vi "open standards data 2.vi"(11 "file path":path) -> (0 "canceled":bool, 1 "standard cluster":T1={"Description"="", "Setup"={"integration time"=0.5, "rinse time"=10.0, "sample time"=10.0, "sample type"=0}, "Concentrations"=[], "Absorbance"=[], "Analyst"="", "Concentration units"="", "Good"=[]} {"Absorbance" format="%.2e"; "Concentrations" format="%.3e"; "Setup"."sample type" items=["Sample Cuvet", "Sipper Cell", "No Dialog"]; "Setup"."sample time" min=0.0 max=100.0 step=1.0 format="%.1f"; "Setup"."rinse time" min=0.0 max=100.0 step=1.0 format="%.1f"; "Setup"."integration time" format="%.1f"}, 3 "new file path":path)   [LabVIEW 2015]
uses:
  standard cluster.ctl
  settings.ctl
  file/file action.ctl
panel:
  out "error out":errorcluster
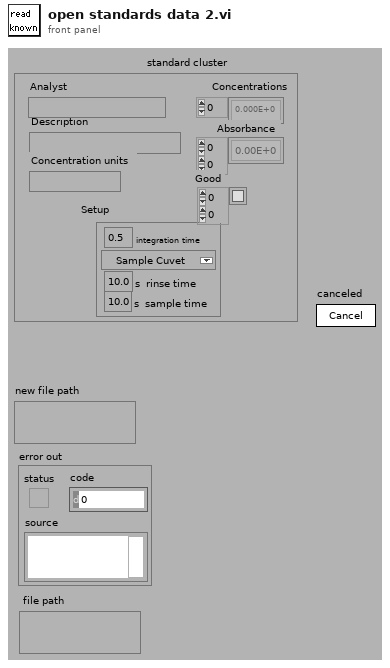
[diagram p1: front panel]
types:
  T1 = typedef "standard cluster.ctl" = cluster{"Description":string, "Setup":T2, "Concentrations":dbl[], "Absorbance":dbl[][], "Analyst":string, "Concentration units":string, "Good":bool[][]}
  T2 = typedef "settings.ctl" = cluster{"integration time":sgl, "rinse time":dbl[unit], "sample time":dbl[unit], "sample type":u16}
  T3 = typedef "file action.ctl" = enum16{"Save", "Open"}
  T4 = enum16{"open", "open or create", "create or replace", "create", "open (read only)"}
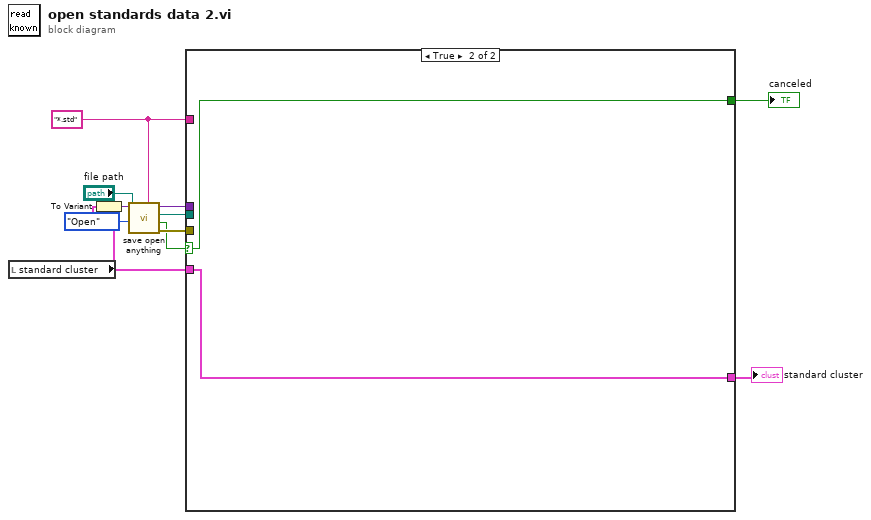
[diagram p0: block diagram]
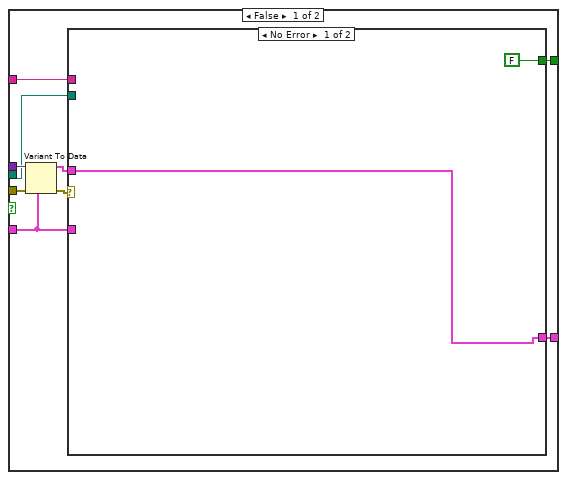
[diagram p2: hidden frame]
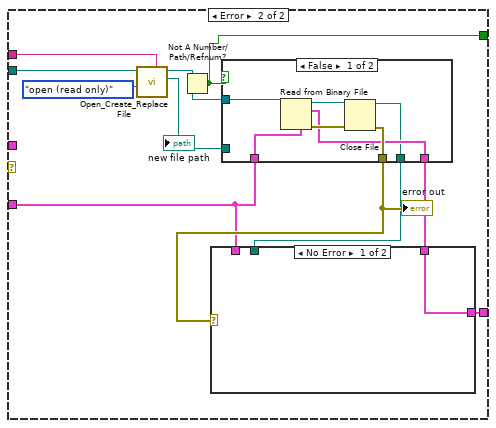
[diagram p3: hidden frame]
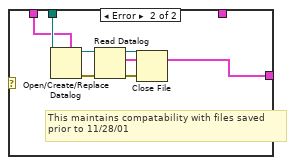
[diagram p4: hidden frame]
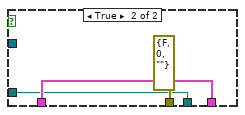
[diagram p5: hidden frame]
diagram:
  w4 = "*.std" ("pattern")
  n1 = local read "standard cluster"() -> (w6:T1)
  n2 = To Variant(anything=w6) -> (Variant=w10:variant)
  n3 = call "save open anything.vi"("Variant"=w10, "file path"="file path", "Action"=file_action."Open", "pattern"=w4) -> ("Variant out"=w8:variant, "new file path"=w5:path, "canceled"=w2:bool, "error out"=w7:errorcluster)  [unwired: 3 in]
  n4 = case shown="True" w2 {
    selector: w2 -> [_ w52]
    tunnel: [w20 w53] -> w11
    tunnel: w8 -> [w19 _]
    tunnel: w7 -> [w18 _]
    tunnel: w6 -> [w17 w53]
    tunnel: w5 -> [w14 _]
    tunnel: w4 -> [w13 _]
    tunnel: [w12 w52] -> w1
    frame False {
      n5 = Variant To Data(error in=w18, type=w17, Variant=w19) -> (data=w15:T1, error out=w16:errorcluster)
      n6 = case shown="No Error" w16 {
        tunnel: [w22 w30] -> w20
        tunnel: w13 -> [_ w26]
        tunnel: w17 -> [_ w25]
        tunnel: w15 -> [w22 _]
        tunnel: w14 -> [_ w24]
        tunnel: [FALSE w23] -> w12
        frame No Error {
        }
        frame Error {
          n7 = call <vilib>:"Open_Create_Replace File.vi"("pattern"=w26, "function (open:0)"=T4."open (read only)", "file path"=w24) -> ("new file path"=w27:path, "refnum"=w32:refnum<file>)  [unwired: 5 in, 2 out]
          "new file path" <- w27
          n8 = Not A Number/Path/Refnum?(number/path/refnum=w32) -> (NaN/Path/Refnum?=w23:bool)
          n9 = case shown="False" w23 {
            tunnel: w32 -> [w46 _]
            tunnel: w25 -> [w45 w50]
            tunnel: [w44 errorcluster {"status"=FALSE, "code"=0, "source"=""} ("error out")] -> w31
            tunnel: [w43 w50] -> w29
            tunnel: [w42 w49] -> w28
            tunnel: w27 -> [_ w49]
            frame False {
              n10 = Read from Binary File(5:w45, 11:w46) -> (0:w47:errorcluster, 2:w43:T1, 3:w48:refnum<file>)  [unwired: 4 in, 1 out]
              n11 = Close File(refnum=w48, error in=w47) -> (path=w42:path, error out=w44:errorcluster)
            }
            frame True {
            }
          }
          "error out" <- w31
          n12 = case shown="No Error" w31 {
            tunnel: [w34 w41] -> w30
            tunnel: w29 -> [w34 _]
            tunnel: w28 -> [_ w36]
            tunnel: w25 -> [_ w35]
            frame No Error {
            }
            frame Error {
              # "This maintains compatability with files saved \nprior to 11/28/01"
              n13 = Open/Create/Replace Datalog(5:w35, 11:w36) -> (0:w38:errorcluster, 3:w39:refnum<k1>)  [unwired: 4 in, 1 out]
              n14 = Read Datalog(4:w38, 7:w39) -> (0:w37:errorcluster, 2:w41:T1, 3:w40:refnum<k1>)  [unwired: 1 in]
              n15 = Close File(refnum=w40, error in=w37) -> ()  [unwired: 2 out]
            }
          }
        }
      }
    }
    frame True {
    }
  }
  "standard cluster" <- w11
  "canceled" <- w1
